vi "Lock_RH_v2.vi"() -> ()   [LabVIEW 2019]
uses:
  <vilib>/Analysis/baseanly.llb/Mean (DBL).vi
  Components/DeltaRamp_globals.vi
  Components/B_Globals.vi
  Components/Global 2.vi
  <vilib>/Analysis/NI_AALBase.lvlib
panel:
  out "R2":dbl
  in  "RW Delay 2":i32=50
  in  "L2_use":bool
  in  "L1_use":bool
  in  "L2":refnum<visa-resource-name>="GPIB1::20::INSTR"
  in  "L1":refnum<visa-resource-name>="GPIB1::20::INSTR"
  in  "Freq":dbl=71.34 format="%#_6e"
  out "B_set [T]":dbl
  in  "Reading Delay [ms]":i32=100 min=5
  in  "RW Delay":i32=50
  out "Exec Time [ms]":u32
  in  "B/T":bool
  in  "Smart Avs":bool=TRUE
  in  "Points":dbl=1.0
  out "PpP":dbl
  in  "Combo Box":string(combo)
  in  "Save":bool
  in  "Abort Delta":bool
  out "B [T]":dbl=0.49837
  in  "Arm":bool
  in  "Measure":bool
  in  "I_Max":dbl=0.00055
  out "T":cluster{"X":dbl[], "Y":dbl[]}[](graph)=[{"X"=[0.48596000000030654, 0.48632999999976745, 0.4888800000004717, 0.4914299999991856, 0.49799999999988437, 0.49837000000048626, 0.49799999999964834, 0.49764000000059827, 0.4972699999998548, 0.49799999999964706, 0.4976400000005962, 0.4979999999996451, 0.49764000000114167, 0.4987299999995217, 0.49837000000048276, 0.4979999999996453, 0.49764000000060443, 0.4980000000000499, 0.4983700000004744, 0.4979999999996602, 0.4983700000001006, 0.4979999999996734, 0.49764000000018094, 0.4979999999996305, 0.4976400000006558, 0.4979999999996311, 0.4976399999998779, 0.49799999999967304, 0.4983699999999628, 0.49799999999964784, 0.49764000000002906, 0.4983699999999084, 0.49799999999967276, 0.498370000000109, 0.4979999999996426, 0.4983700000001016, 0.4979999999996246, 0.4983700000001098, 0.4979999999996428, 0.4976400000006453], "Y"=[nan, nan, nan, nan, nan, nan, nan, nan, nan, nan, nan, nan, nan, nan, nan, nan, nan, nan, nan, nan, nan, nan, nan, nan, nan, nan, nan, nan, nan, nan, nan, nan, nan, nan, nan, nan, nan, nan, nan, nan]}] caption="XY Graph"
  in  "Reset":bool
  out "Spl T [K]":dbl=6.1992
  out "R1 [Ohm]":dbl=nan
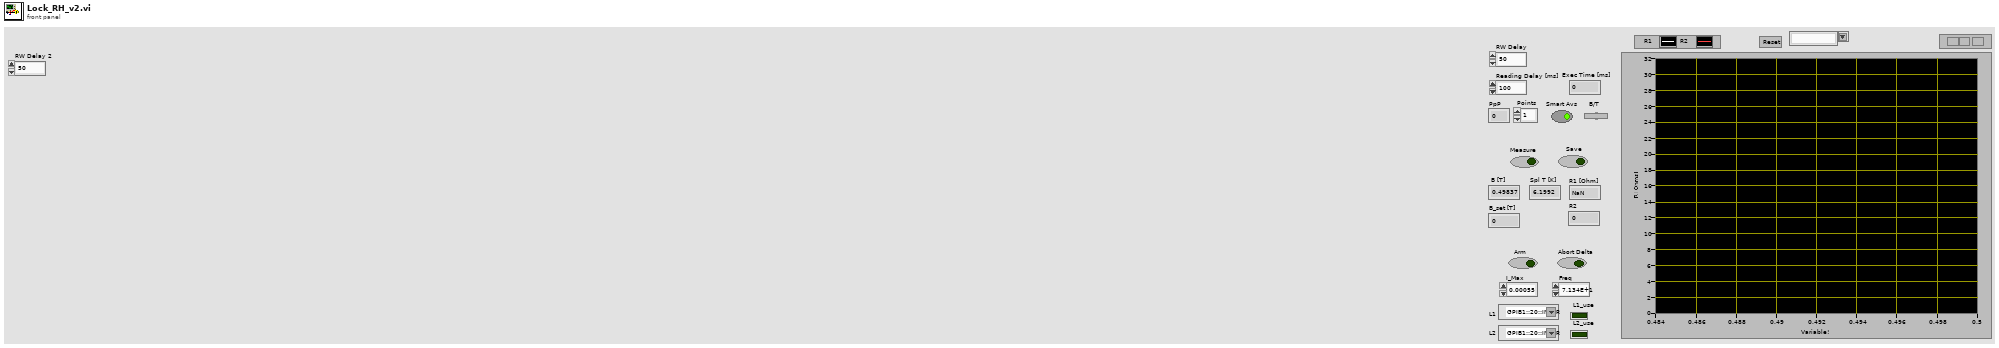
[diagram p1: front panel]
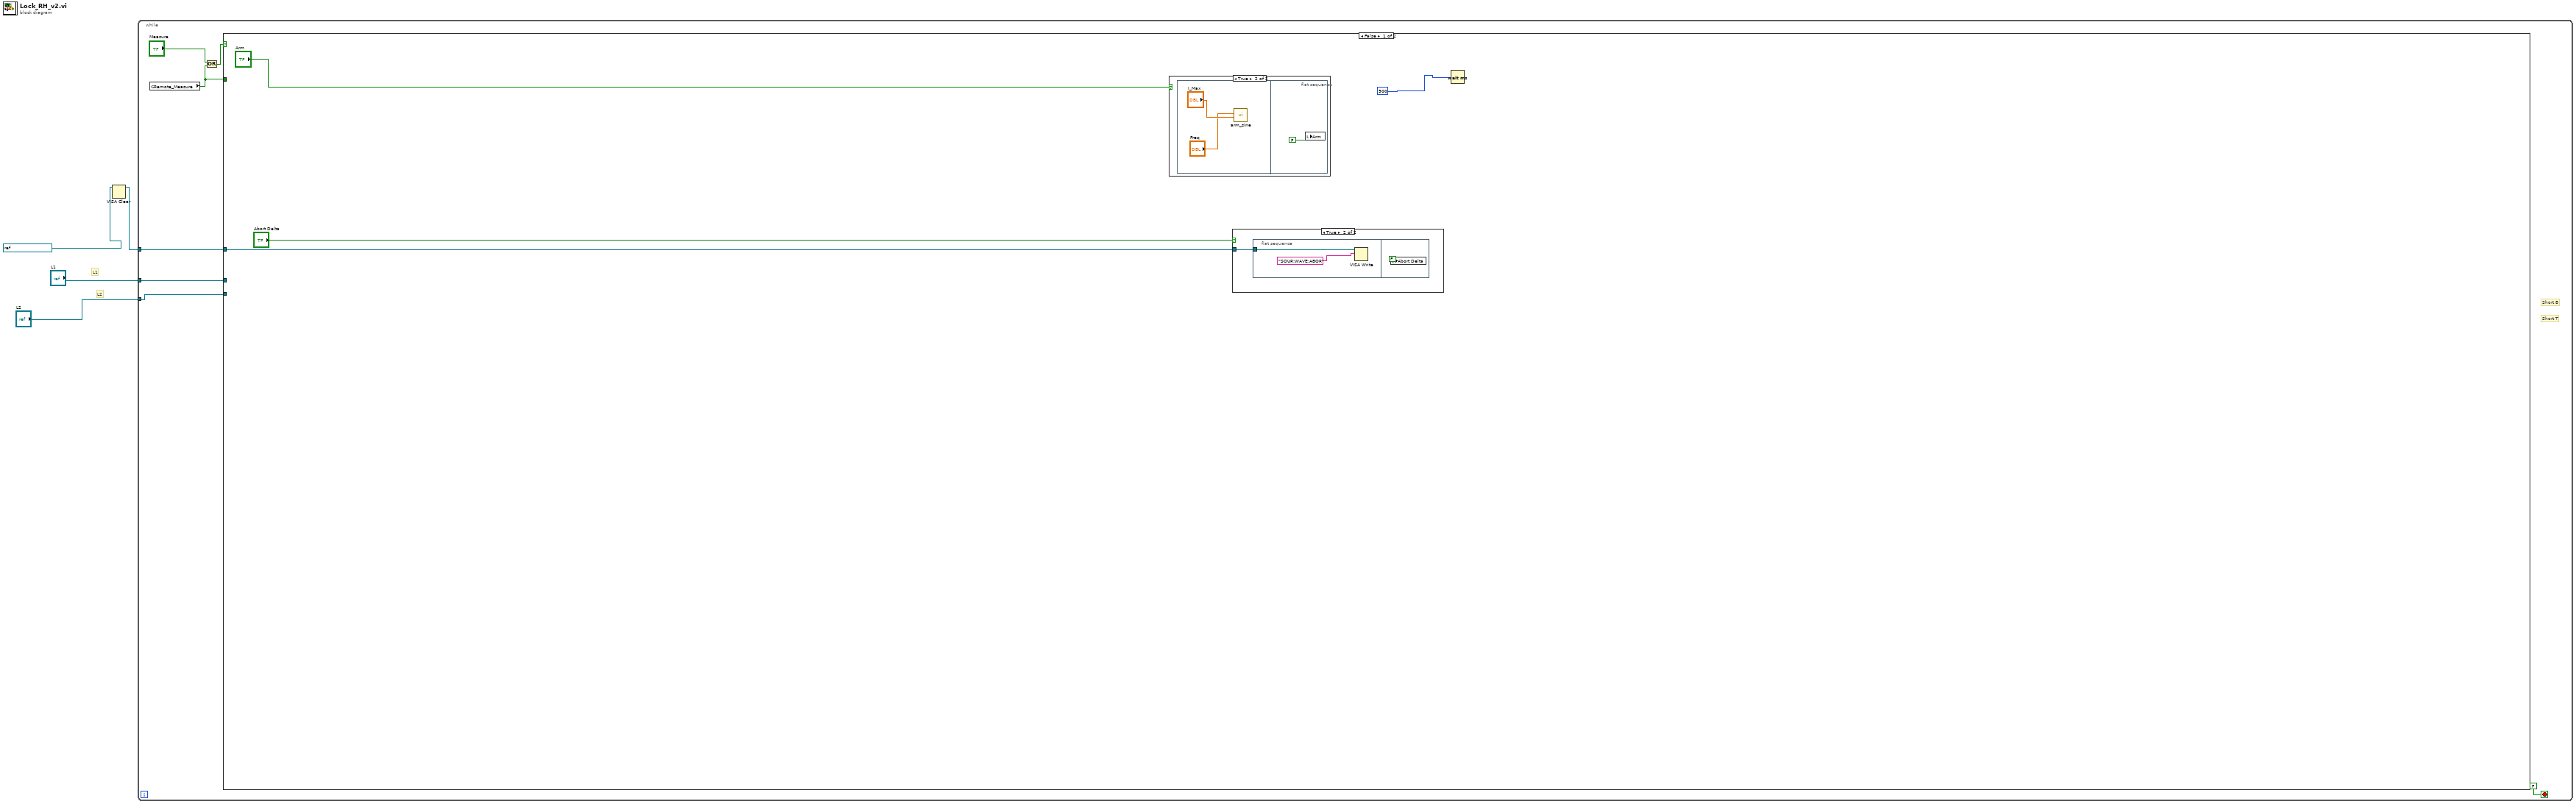
[diagram p0: block diagram]
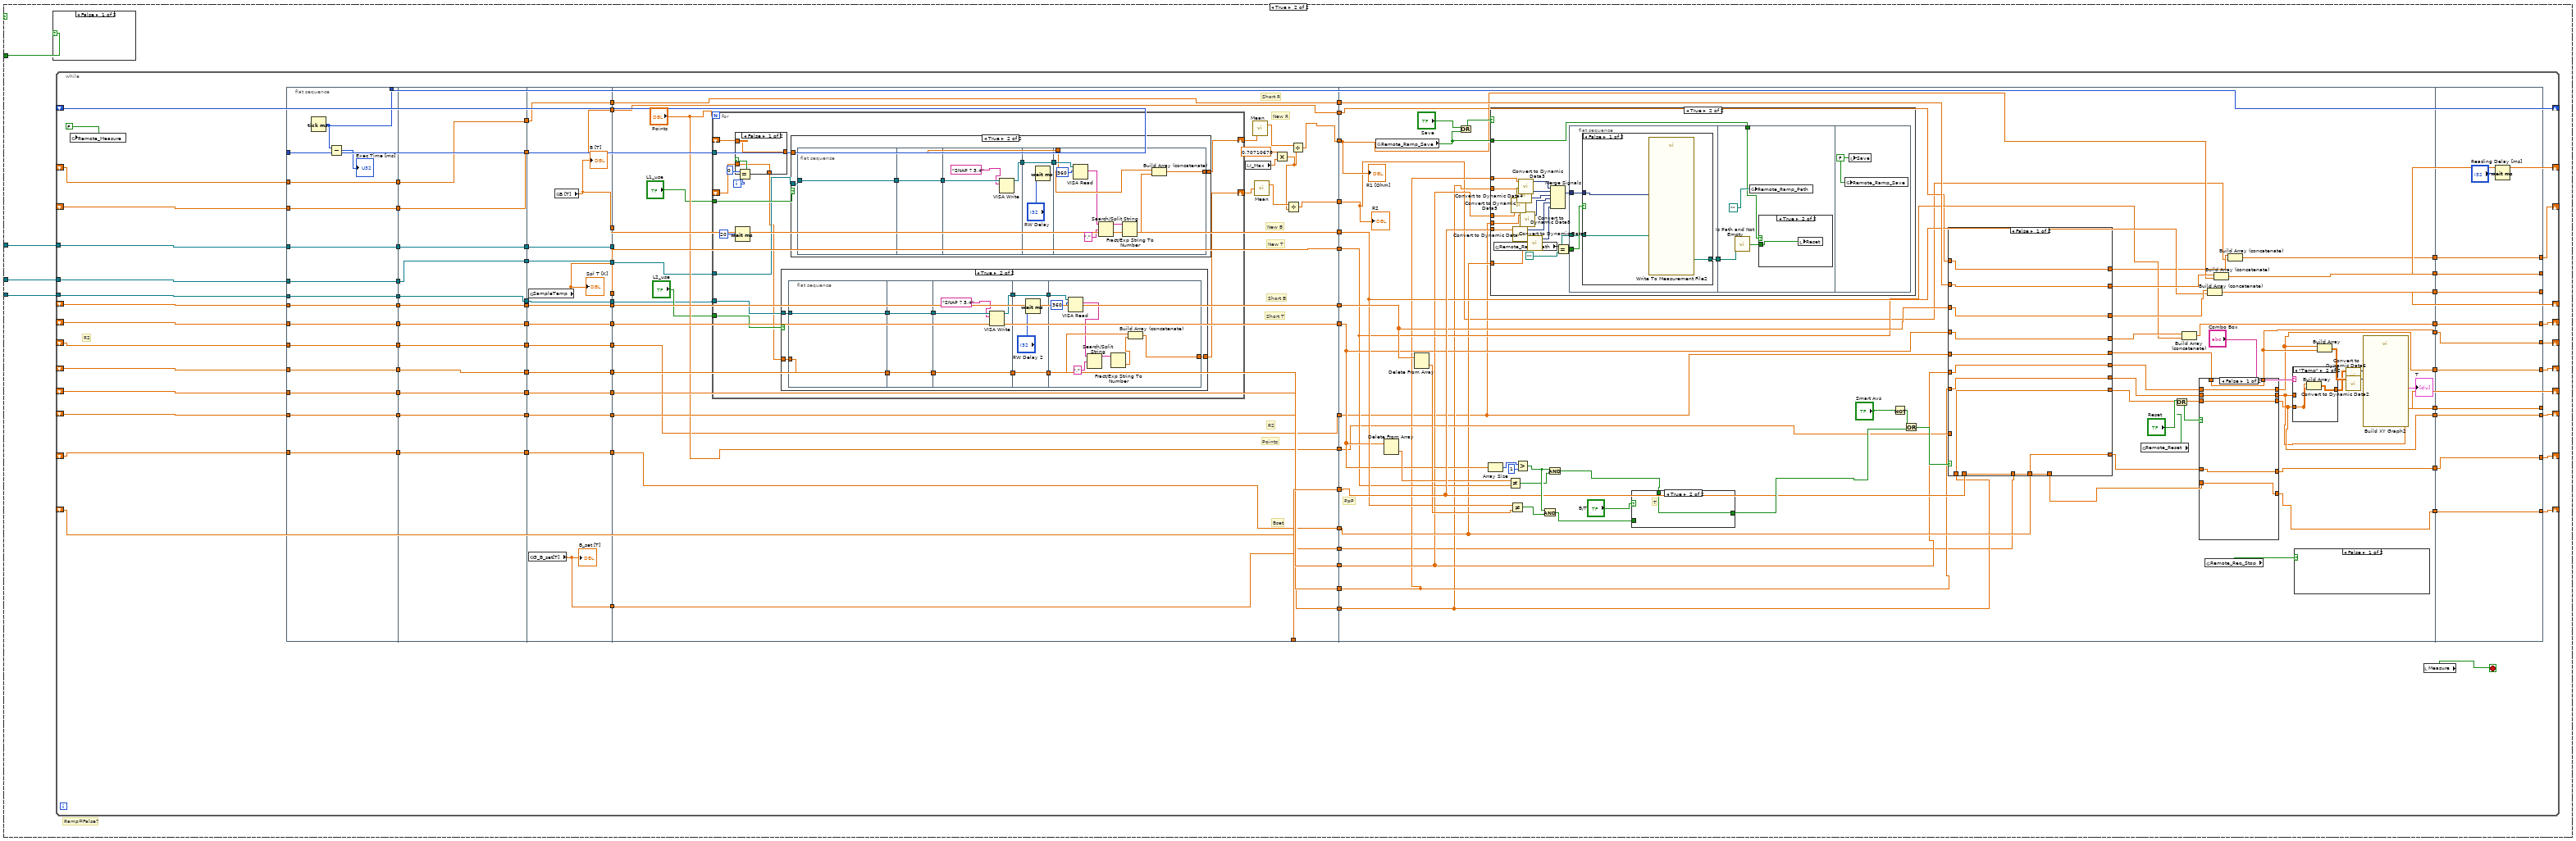
[diagram p4: hidden frame]
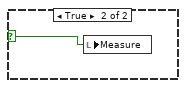
[diagram p5: hidden frame]
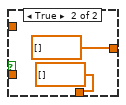
[diagram p8: hidden frame]
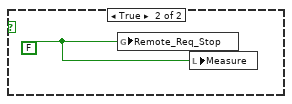
[diagram p10: hidden frame]
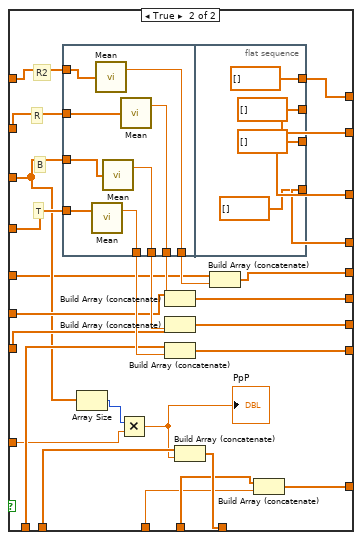
[diagram p11: hidden frame]
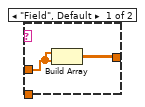
[diagram p12: hidden frame]
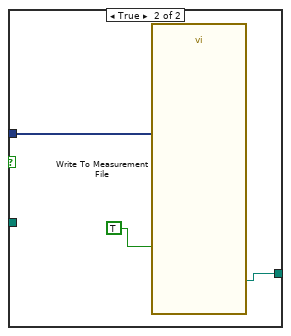
[diagram p14: hidden frame]
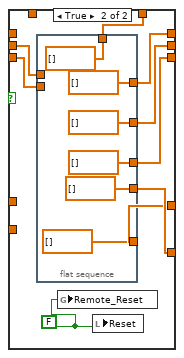
[diagram p16: hidden frame]
diagram:
  # "L2"
  # "L1"
  n1 = VISA Clear(VISA resource name=refnum<visa-resource-name> "GPIB1::20::INSTR" ("Keithley")) -> (VISA resource name out=w4:refnum<visa-resource-name>)  [unwired: 1 in, 1 out]
  n2 = while {
    tunnel: w4 -> [w10]
    tunnel: "L1" -> [w6]
    tunnel: "L2" -> [w5]
    stop <- FALSE stop-if-true
    # "Short T"
    # "Short B"
    n3 = global read "DeltaRamp_globals.vi" "Remote_Measure"() -> (w7:bool)
    n4 = Or(x="Measure", y=w7) -> (x .or. y?=w9:bool)
    n5 = case shown="False" w9 {
      tunnel: w10 -> [w13 w26]
      tunnel: w7 -> [_ w25]
      tunnel: w6 -> [_ w24]
      tunnel: w5 -> [_ w23]
      frame False {
        n6 = case shown="True" "Arm" {
          frame False {
          }
          frame True {
            n7 = flat-sequence {
              frame #0 {
                n8 = call "arm_sine.vi"("Peak Amp"="I_Max", "Freq"="Freq") -> ()  [unwired: 10 in]
              }
              frame #1 {
                n9 = local write "Arm"(FALSE) -> ()
              }
            }
          }
        }
        n10 = case shown="True" "Abort Delta" {
          tunnel: w13 -> [_ w16]
          frame False {
          }
          frame True {
            n11 = flat-sequence {
              tunnel: w16 -> [w18]
              frame #0 {
                n12 = VISA Write(VISA resource name=w18, write buffer="SOUR:WAVE:ABOR") -> ()  [unwired: 1 in, 3 out]
              }
              frame #1 {
                n13 = local write "Abort Delta"(FALSE) -> ()
              }
            }
          }
        }
        n14 = Wait (ms)(milliseconds to wait=500) -> ()  [unwired: 1 out]
      }
      frame True {
        # "Ramp=False?"
        n15 = case shown="False" w25 {
          selector: w25 -> [_ w27]
          frame False {
          }
          frame True {
            n16 = local write "Measure"(w27) -> ()
          }
        }
        n17 = while {
          shift-right: [w70] -> _
          shift-left: _ -> [w77]
          shift-right: [w89] -> _
          shift-left: _ -> [w94]
          tunnel: w26 -> [w113]
          shift-right: [w87] -> _
          shift-left: _ -> [w100]
          shift-right: [w69] -> _
          shift-left: _ -> [w81]
          shift-right: [w71] -> _
          shift-left: _ -> [w86]
          shift-right: [w88] -> _
          shift-left: _ -> [w104]
          shift-right: [w114] -> _
          shift-left: _ -> [w115]
          shift-right: [w117] -> _
          shift-left: _ -> [w118]
          shift-right: [w53] -> _
          shift-left: _ -> [w58]
          tunnel: w24 -> [w50]
          tunnel: w23 -> [w49]
          shift-right: [w35] -> _
          shift-left: _ -> [w40]
          shift-right: [w33] -> _
          shift-left: _ -> [w31]
          stop <- w60 stop-if-true
          # "R2"
          n18 = global write "DeltaRamp_globals.vi" "Remote_Measure"(FALSE) -> ()
          n19 = flat-sequence {
            tunnel: w118 -> [w134]
            tunnel: [w132] -> w117
            tunnel: w113 -> [w131]
            tunnel: [w131] -> w110
            tunnel: w104 -> [w130]
            tunnel: [w130] -> w103
            tunnel: w100 -> [w129]
            tunnel: [w129] -> w97
            tunnel: w94 -> [w128]
            tunnel: [w128] -> w92
            tunnel: w86 -> [w127]
            tunnel: [w127] -> w83
            tunnel: [w126] -> w82
            tunnel: w81 -> [w126]
            tunnel: [w125] -> w78
            tunnel: w77 -> [w125]
            tunnel: [w124] -> w59
            tunnel: w58 -> [w124]
            tunnel: w50 -> [w123]
            tunnel: w49 -> [w122]
            tunnel: [w123] -> w48
            tunnel: [w122] -> w47
            tunnel: [w121] -> w41
            tunnel: w40 -> [w121]
            tunnel: [w120] -> w32
            tunnel: w31 -> [w120]
            tunnel: [w146] -> w111
            tunnel: w110 -> [w146]
            tunnel: w103 -> [w145]
            tunnel: [w145] -> w102
            tunnel: [w144] -> w98
            tunnel: w97 -> [w144]
            tunnel: [w143] -> w93
            tunnel: w92 -> [w143]
            tunnel: [w142] -> w84
            tunnel: w83 -> [w142]
            tunnel: w82 -> [w141]
            tunnel: [w141] -> w79
            tunnel: w78 -> [w140]
            tunnel: [w140] -> w75
            tunnel: w59 -> [w139]
            tunnel: [w139] -> w56
            tunnel: w48 -> [w138]
            tunnel: w47 -> [w137]
            tunnel: [w138] -> w45
            tunnel: [w137] -> w43
            tunnel: w41 -> [w136]
            tunnel: [w136] -> w39
            tunnel: w32 -> [w135]
            tunnel: [w135] -> w29
            tunnel: [w161] -> w112
            tunnel: w111 -> [w161]
            tunnel: [w160] -> w108
            tunnel: [w159] -> w106
            tunnel: w102 -> [w158]
            tunnel: [w158] -> w101
            tunnel: [w157] -> w99
            tunnel: w98 -> [w157]
            tunnel: w93 -> [w156]
            tunnel: [w156] -> w91
            tunnel: [w155] -> w85
            tunnel: w84 -> [w155]
            tunnel: [w154] -> w80
            tunnel: w79 -> [w154]
            tunnel: [w153] -> w76
            tunnel: w75 -> [w153]
            tunnel: [w152] -> w57
            tunnel: w56 -> [w152]
            tunnel: [w151] -> w52
            tunnel: [w150] -> w46
            tunnel: w45 -> [w150]
            tunnel: [w149] -> w44
            tunnel: w43 -> [w149]
            tunnel: w39 -> [w148]
            tunnel: [w148] -> w37
            tunnel: [w147] -> w30
            tunnel: w29 -> [w147]
            tunnel: [w188] -> w116
            tunnel: w115 -> [w188]
            tunnel: w112 -> [w187]
            tunnel: [w166] -> w109
            tunnel: w108 -> [w186]
            tunnel: [w186] -> w107
            tunnel: w106 -> [w185]
            tunnel: [w185] -> w105
            tunnel: w101 -> [w184]
            tunnel: w99 -> [w183]
            tunnel: [w184] -> w96
            tunnel: [w183] -> w95
            tunnel: w91 -> [w182]
            tunnel: [w182] -> w90
            tunnel: w85 -> [w181]
            tunnel: w80 -> [w180]
            tunnel: w76 -> [w179]
            tunnel: [w181] -> w74
            tunnel: [w180] -> w73
            tunnel: [w179] -> w72
            tunnel: ["Points"] -> w68
            tunnel: w57 -> [w177]
            tunnel: [w177] -> w55
            tunnel: w52 -> [w176]
            tunnel: [w176] -> w51
            tunnel: w46 -> [w172]
            tunnel: w44 -> [w173]
            tunnel: [w165] -> w42
            tunnel: [w168] -> w38
            tunnel: w37 -> [w168]
            tunnel: w30 -> [w167]
            tunnel: [w167] -> w28
            tunnel: w116 -> [w298]
            tunnel: w109 -> [w290]
            tunnel: w107 -> [w289]
            tunnel: w105 -> [w285]
            tunnel: w96 -> [w294]
            tunnel: w95 -> [w288]
            tunnel: w90 -> [w293]
            tunnel: w74 -> [w277]
            tunnel: w73 -> [w276]
            tunnel: w72 -> [w275]
            tunnel: w68 -> [w281]
            tunnel: [w282] -> w67
            tunnel: [w291] -> w66
            tunnel: [w287] -> w65
            tunnel: [w286] -> w64
            tunnel: [w264] -> w63
            tunnel: [w284] -> w62
            tunnel: [w283] -> w61
            tunnel: w55 -> [w278]
            tunnel: [w280] -> w54
            tunnel: w51 -> [w274]
            tunnel: w42 -> [w270]
            tunnel: w38 -> [w273]
            tunnel: [w271] -> w36
            tunnel: [w266] -> w34
            tunnel: w28 -> [w268]
            tunnel: [w441] -> w69
            tunnel: [w442] -> w70
            tunnel: [w443] -> w71
            tunnel: [w444] -> w87
            tunnel: [w445] -> w88
            tunnel: [w446] -> w89
            tunnel: [w447] -> w114
            tunnel: w67 -> [w447]
            tunnel: w66 -> [w446]
            tunnel: w65 -> [w445]
            tunnel: w64 -> [w444]
            tunnel: w63 -> [w443]
            tunnel: w62 -> [w442]
            tunnel: w61 -> [w441]
            tunnel: w54 -> [w439]
            tunnel: [w439] -> w53
            tunnel: [w438] -> w35
            tunnel: w36 -> [w438]
            tunnel: w34 -> [w437]
            tunnel: [w437] -> w33
            frame #0 {
              n20 = Tick Count (ms)() -> (millisecond timer value=w132:u32)
              n21 = Subtract(x=w132, y=w134) -> (x-y=→"Exec Time [ms]":u32)
            }
            frame #1 {
            }
            frame #2 {
              n22 = global read "Global 2.vi" "SampleTemp"() -> (w159:dbl)
              "Spl T [K]" <- w159
              n23 = global read "B_Globals.vi" "G_B_set[T]"() -> (w151:dbl)
              "B_set [T]" <- w151
              n24 = global read "B_Globals.vi" "B [T]"() -> (w160:dbl)
              "B [T]" <- w160
            }
            frame #3 {
              # "R2"
              # "Bset"
              # "Points"
              # "Short R"
              # "New T"
              # "New B"
              # "Short T"
              # "Short B"
              # "New R"
              n25 = for {
                N: "Points" -> [_]
                tunnel: w187 -> [_]
                shift-right: [w194] -> w189
                shift-left: _ -> [w200]
                tunnel: "L2_use" -> [w199]
                tunnel: "L1_use" -> [w198]
                tunnel: w173 -> [w197]
                tunnel: w172 -> [w196]
                shift-right: [w191] -> w171
                shift-left: _ -> [w193]
                i -> [w201]
                n26 = Wait (ms)(milliseconds to wait=20) -> ()  [unwired: 1 out]
                n27 = Equal?(x=0, y=w201) -> (x = y?=w203:bool)
                n28 = case shown="False" w203 {
                  tunnel: [w259 dbl[] [] ("Numeric")] -> w195
                  tunnel: w200 -> [w259 _]
                  tunnel: w193 -> [w258 _]
                  tunnel: [w258 dbl[] [] ("Numeric")] -> w192
                  frame False {
                  }
                  frame True {
                  }
                }
                n29 = case shown="True" w199 {
                  tunnel: w197 -> [_ w234]
                  tunnel: w192 -> [w227 w233]
                  tunnel: [w227 w228] -> w191
                  frame False {
                  }
                  frame True {
                    n30 = flat-sequence {
                      tunnel: w234 -> [w240]
                      tunnel: [w240] -> w238
                      tunnel: w233 -> [w239]
                      tunnel: [w239] -> w231
                      tunnel: w238 -> [w242]
                      tunnel: [w242] -> w237
                      tunnel: [w241] -> w232
                      tunnel: w231 -> [w241]
                      tunnel: [w245] -> w236
                      tunnel: w237 -> [w246]
                      tunnel: w232 -> [w243]
                      tunnel: [w243] -> w229
                      tunnel: [w248] -> w235
                      tunnel: w236 -> [w248]
                      tunnel: [w247] -> w230
                      tunnel: w229 -> [w247]
                      tunnel: w235 -> [w256]
                      tunnel: w230 -> [w255]
                      tunnel: [w254] -> w228
                      frame #0 {
                      }
                      frame #1 {
                      }
                      frame #2 {
                        n31 = VISA Write(VISA resource name=w246, write buffer="SNAP ? 3,4") -> (VISA resource name out=w245:refnum<visa-resource-name>)  [unwired: 1 in, 2 out]
                      }
                      frame #3 {
                        n32 = Wait (ms)(milliseconds to wait="RW Delay 2") -> ()  [unwired: 1 out]
                      }
                      frame #4 {
                        n33 = VISA Read(VISA resource name=w256, byte count=u32 360) -> (read buffer=w252:string)  [unwired: 1 in, 3 out]
                        n34 = Search/Split String(string=w252, search string/char (-)=",") -> (substring before match=w251:string)  [unwired: 1 in, 2 out]
                        n35 = Fract/Exp String To Number(string=w251) -> (number=w253:dbl)  [unwired: 1 in, 3 out]
                        n36 = Build Array (concatenate)(w255, w253) -> (w254:dbl[])
                      }
                    }
                  }
                }
                n37 = case shown="True" w198 {
                  tunnel: w196 -> [_ w207]
                  tunnel: w195 -> [w204 w206]
                  tunnel: [w204 w205] -> w194
                  frame False {
                  }
                  frame True {
                    n38 = flat-sequence {
                      tunnel: w207 -> [w212]
                      tunnel: [w212] -> w211
                      tunnel: w211 -> [w213]
                      tunnel: [w213] -> w210
                      tunnel: [w215] -> w209
                      tunnel: w210 -> [w216]
                      tunnel: [w217] -> w208
                      tunnel: w209 -> [w217]
                      tunnel: w208 -> [w225]
                      tunnel: w206 -> [w224]
                      tunnel: [w223] -> w205
                      frame #0 {
                      }
                      frame #1 {
                      }
                      frame #2 {
                        n39 = VISA Write(VISA resource name=w216, write buffer="SNAP ? 3,4") -> (VISA resource name out=w215:refnum<visa-resource-name>)  [unwired: 1 in, 2 out]
                      }
                      frame #3 {
                        n40 = Wait (ms)(milliseconds to wait="RW Delay") -> ()  [unwired: 1 out]
                      }
                      frame #4 {
                        n41 = VISA Read(VISA resource name=w225, byte count=u32 360) -> (read buffer=w221:string)  [unwired: 1 in, 3 out]
                        n42 = Search/Split String(string=w221, search string/char (-)=",") -> (substring before match=w220:string)  [unwired: 1 in, 2 out]
                        n43 = Fract/Exp String To Number(string=w220) -> (number=w219:dbl)  [unwired: 1 in, 3 out]
                        n44 = Build Array (concatenate)(w224, w219) -> (w223:dbl[])
                      }
                    }
                  }
                }
              }
              n45 = local read "I_Max"() -> (w163:dbl)
              n46 = call-poly <vilib>:"Mean.vi"("X"=w189) -> ("mean"=w170:dbl)  [unwired: 1 out]
              n47 = call-poly <vilib>:"Mean.vi"("X"=w171) -> ("mean"=w169:dbl)  [unwired: 1 out]
              n48 = Multiply(x=0.70710678, y=w163) -> (x*y=w164:dbl)
              n49 = Divide(x=w169, y=w164) -> (x/y=w165:dbl)
              n50 = Divide(x=w170, y=w164) -> (x/y=w166:dbl)
            }
            frame #4 {
              # "PpP"
              n51 = global read "DeltaRamp_globals.vi" "Remote_Ramp_Save"() -> (w310:bool)
              n52 = Delete From Array(array=w288) -> (deleted portion=w296:dbl)  [unwired: 2 in, 1 out]
              n53 = Delete From Array(array=w294) -> (deleted portion=w295:dbl)  [unwired: 2 in, 1 out]
              n54 = Or(x="Save", y=w310) -> (x .or. y?=w305:bool)
              n55 = Array Size(array=w288) -> (size(s)=w315:i32)
              n56 = case shown="True" w305 {
                tunnel: w310 -> [_ w394]
                tunnel: w298 -> [_ w393]
                tunnel: w278 -> [_ w388]
                tunnel: w277 -> [_ w391]
                tunnel: w276 -> [_ w390]
                tunnel: w275 -> [_ w389]
                tunnel: w268 -> [_ w382]
                frame False {
                }
                frame True {
                  n57 = global read "DeltaRamp_globals.vi" "Remote_Ramp_Path"() -> (w396:path)
                  n58 = call "Convert to Dynamic Data5"("Array"=w391) -> ("Dynamic Data Type"=w384:dynamicdata)  [unwired: 3 in]
                  n59 = call "Convert to Dynamic Data"("Array"=w393) -> ("Dynamic Data Type"=w392:dynamicdata)  [unwired: 3 in]
                  n60 = call "Convert to Dynamic Data4"("Array"=w389) -> ("Dynamic Data Type"=w385:dynamicdata)  [unwired: 3 in]
                  n61 = call "Convert to Dynamic Data3"("Array"=w390) -> ("Dynamic Data Type"=w386:dynamicdata)  [unwired: 3 in]
                  n62 = call "Convert to Dynamic Data8"("Array"=w382) -> ("Dynamic Data Type"=w383:dynamicdata)  [unwired: 3 in]
                  n63 = call "Convert to Dynamic Data7"("Array"=w388) -> ("Dynamic Data Type"=w387:dynamicdata)  [unwired: 3 in]
                  n64 = Merge Signals(w386, w385, w384, w383, w392, w387) -> (w399:dynamicdata)
                  n65 = Equal?(x=w396, y=path "") -> (x = y?=w397:bool)
                  n66 = flat-sequence {
                    tunnel: w399 -> [w403]
                    tunnel: w397 -> [w402]
                    tunnel: w396 -> [w401]
                    tunnel: [w400] -> w395
                    tunnel: w395 -> [w412]
                    tunnel: w394 -> [w411]
                    frame #0 {
                      n67 = case shown="False" w402 {
                        tunnel: w403 -> [w406 w408]
                        tunnel: w401 -> [w405 _]
                        tunnel: [w404 w407] -> w400
                        frame False {
                          n68 = call "Write To Measurement File2"("Signals"=w406, "Filename"=w405) -> ("Filename Out"=w404:path)  [unwired: 15 in, 2 out]
                        }
                        frame True {
                          n69 = call "Write To Measurement File"("Signals"=w408, "Reset"=TRUE) -> ("Filename Out"=w407:path)  [unwired: 15 in, 2 out]
                        }
                      }
                    }
                    frame #1 {
                      n70 = call <vilib>:"Is Path and Not Empty.vi"("path"=w412) -> ("Is Path and Not Empty?"=w410:bool)  [unwired: 4 in]
                      n71 = global write "DeltaRamp_globals.vi" "Remote_Ramp_Path"(path "") -> ()
                      n72 = case shown="True" w411 {
                        tunnel: w410 -> [_ w414]
                        frame False {
                        }
                        frame True {
                          n73 = local write "Reset"(w414) -> ()
                        }
                      }
                    }
                    frame #2 {
                      w415 = FALSE
                      n74 = global write "DeltaRamp_globals.vi" "Remote_Ramp_Save"(w415) -> ()
                      n75 = local write "Save"(w415) -> ()
                    }
                  }
                }
              }
              n76 = Not Equal?(x=w296, y=w285) -> (x != y?=w316:bool)
              n77 = Not Equal?(x=w289, y=w295) -> (x != y?=w319:bool)
              n78 = Greater?(x=w315, y=1) -> (0:w318:bool)
              n79 = And(x=w318, y=w319) -> (x .and. y?=w320:bool)
              n80 = And(x=w318, y=w316) -> (x .and. y?=w321:bool)
              n81 = case shown="True" "B/T" {
                tunnel: w320 -> [w325 _]
                tunnel: w321 -> [_ w326]
                tunnel: [w325 w326] -> w322
                frame False {
                  # "B"
                }
                frame True {
                  # "T"
                }
              }
              n82 = Not(x="Smart Avs") -> (.not. x?=w312:bool)
              n83 = Or(x=w312, y=w322) -> (x .or. y?=w313:bool)
              n84 = case shown="False" w313 {
                tunnel: [w336 w365] -> w324
                tunnel: [w334 w364] -> w292
                tunnel: [w335 w351] -> w323
                tunnel: [w331 w362] -> w301
                tunnel: [w333 w361] -> w302
                tunnel: [w332 w359] -> w303
                tunnel: [w337 w357] -> w297
                tunnel: w298 -> [w337 w356]
                tunnel: w294 -> [w336 w347]
                tunnel: w288 -> [w335 w352]
                tunnel: w293 -> [w334 w353]
                tunnel: w277 -> [w333 w350]
                tunnel: w276 -> [w331 w349]
                tunnel: w275 -> [w332 w348]
                tunnel: w281 -> [_ w346]
                tunnel: w278 -> [w330 w345]
                tunnel: [w330 w344] -> w279
                tunnel: w274 -> [_ w343]
                tunnel: w273 -> [w329 w342]
                tunnel: [w329 w341] -> w272
                tunnel: [w328 w339] -> w269
                tunnel: w268 -> [w328 w338]
                frame False {
                }
                frame True {
                  # "R2"
                  # "T"
                  # "B"
                  # "R"
                  n85 = flat-sequence {
                    tunnel: [w372] -> w363
                    tunnel: [w371] -> w358
                    tunnel: [w373] -> w360
                    tunnel: w353 -> [w370]
                    tunnel: w347 -> [w369]
                    tunnel: w352 -> [w368]
                    tunnel: w342 -> [w367]
                    tunnel: [w366] -> w340
                    tunnel: [dbl[] []] -> w351
                    tunnel: [dbl[] []] -> w365
                    tunnel: [dbl[] []] -> w364
                    tunnel: [dbl[] []] -> w341
                    frame #0 {
                      n86 = call-poly <vilib>:"Mean.vi"("X"=w368) -> ("mean"=w373:dbl)  [unwired: 1 out]
                      n87 = call-poly <vilib>:"Mean.vi"("X"=w367) -> ("mean"=w366:dbl)  [unwired: 1 out]
                      n88 = call-poly <vilib>:"Mean.vi"("X"=w369) -> ("mean"=w372:dbl)  [unwired: 1 out]
                      n89 = call-poly <vilib>:"Mean.vi"("X"=w370) -> ("mean"=w371:dbl)  [unwired: 1 out]
                    }
                    frame #1 {
                    }
                  }
                  n90 = Array Size(array=w347) -> (size(s)=w355:i32)
                  n91 = Multiply(x=w355, y=w346) -> (x*y=w354:dbl)
                  "PpP" <- w354
                  n92 = Build Array (concatenate)(w350, w358) -> (w361:dbl[])
                  n93 = Build Array (concatenate)(w349, w363) -> (w362:dbl[])
                  n94 = Build Array (concatenate)(w348, w360) -> (w359:dbl[])
                  n95 = Build Array (concatenate)(w356, w354) -> (w357:dbl[])
                  n96 = Build Array (concatenate)(w338, w340) -> (w339:dbl[])
                  n97 = Build Array (concatenate)(w345, w343) -> (w344:dbl[])
                }
              }
              n98 = global read "DeltaRamp_globals.vi" "Remote_Reset"() -> (w306:bool)
              n99 = Or(x="Reset", y=w306) -> (x .or. y?=w308:bool)
              n100 = Build Array (concatenate)(w323, w285) -> (w286:dbl[])
              n101 = case shown="False" w308 {
                tunnel: w301 -> [w421 w430]
                tunnel: [w421 w429] -> w283
                tunnel: w303 -> [w420 w428]
                tunnel: [w420 w427] -> w284
                tunnel: [w419 w426] -> w264
                tunnel: w302 -> [w419 _]
                tunnel: [w418 w424] -> w282
                tunnel: w297 -> [w418 _]
                tunnel: [w417 w423] -> w280
                tunnel: w279 -> [w417 _]
                tunnel: w269 -> [w416 _]
                tunnel: [w416 w422] -> w266
                frame False {
                }
                frame True {
                  w425 = FALSE
                  n102 = flat-sequence {
                    tunnel: w430 -> [_]
                    tunnel: w428 -> [_]
                    tunnel: [dbl[] []] -> w427
                    tunnel: [dbl[] []] -> w429
                    tunnel: [dbl[] []] -> w426
                    tunnel: [dbl[] [] ("Numeric")] -> w424
                    tunnel: [dbl[] [] ("Numeric")] -> w423
                    tunnel: [dbl[] [] ("Numeric")] -> w422
                    frame #0 {
                    }
                  }
                  n103 = global write "DeltaRamp_globals.vi" "Remote_Reset"(w425) -> ()
                  n104 = local write "Reset"(w425) -> ()
                }
              }
              n105 = global read "DeltaRamp_globals.vi" "Remote_Req_Stop"() -> (w309:bool)
              n106 = Build Array (concatenate)(w324, w289) -> (w287:dbl[])
              n107 = Build Array (concatenate)(w292, w290) -> (w291:dbl[])
              n108 = Build Array (concatenate)(w272, w270) -> (w271:dbl[])
              n109 = case shown="\"Temp\"" "Combo Box" {
                tunnel: w284 -> [_ w381]
                tunnel: w283 -> [w379 _]
                tunnel: [w378 w380] -> w263
                frame "Field", Default {
                  n110 = Build Array(w379, w379) -> (w378:dbl[][])
                }
                frame "Temp" {
                  n111 = Build Array(w381, w381) -> (w380:dbl[][])
                }
              }
              n112 = case shown="False" w309 {
                frame False {
                }
                frame True {
                  w327 = FALSE
                  n113 = global write "DeltaRamp_globals.vi" "Remote_Req_Stop"(w327) -> ()
                  n114 = local write "Measure"(w327) -> ()
                }
              }
              n115 = Build Array(w264, w266) -> (w267:dbl[][])
              n116 = call "Convert to Dynamic Data6"("2D Array"=w263) -> ("Dynamic Data Type"=w262:dynamicdata)  [unwired: 3 in]
              n117 = call "Convert to Dynamic Data2"("2D Array"=w267) -> ("Dynamic Data Type"=w265:dynamicdata)  [unwired: 3 in]
              n118 = call "Build XY Graph2"("Y Input"=w265, "X Input"=w262) -> ("XY Graph"=→"T":cluster{"X":dbl[], "Y":dbl[]}[])  [unwired: 8 in, 1 out]
              "R1 [Ohm]" <- w290
              "R2" <- w270
            }
            frame #5 {
              n119 = Wait (ms)(milliseconds to wait="Reading Delay [ms]") -> ()  [unwired: 1 out]
            }
          }
          n120 = local read "Measure"() -> (w60:bool)
        }
      }
    }
  }
